vi "BuildTag.vi"(0 "Indent":i8=-1, 2 "tag":string, 3 "value":string, 4 "string in":string) -> (1 "string out":string)   [LabVIEW 2016]
doc: "Builds an XML string with tags"
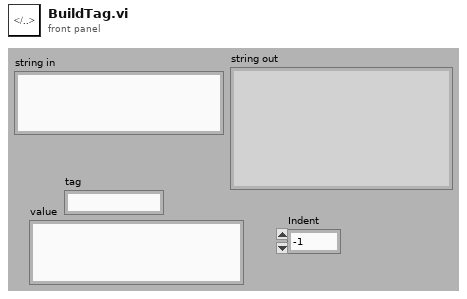
[diagram p1: front panel]
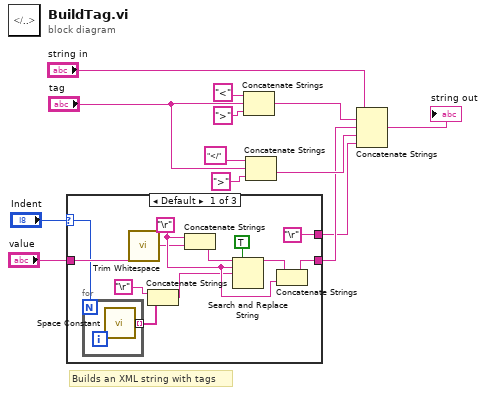
[diagram p0: block diagram]
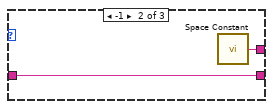
[diagram p2: hidden frame]
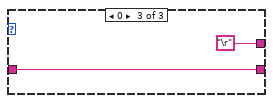
[diagram p3: hidden frame]
diagram:
  # "Builds an XML string with tags"
  n1 = case shown="Default" "Indent" {
    selector: "Indent" -> [w15 _ _]
    tunnel: [w23 w28 w30] -> w5
    tunnel: "value" -> [w20 w28 w30]
    tunnel: ["\r" w27 "\r"] -> w1
    frame Default {
      w22 = "\r"
      n2 = for {
        N: w15 -> [_]
        tunnel: [w26] -> w17 mode=indexing
        n3 = call "Space Constant.vi"() -> ("String"=w26:string)
      }
      n4 = call "Trim Whitespace.vi"("string"=w20) -> ("trimmed string"=w19:string)  [unwired: 1 in]
      n5 = Concatenate Strings("\r", w17) -> (w16:string)
      n6 = Concatenate Strings(w22, w19) -> (w21:string)
      n7 = Search and Replace String(replace all?=TRUE ("replace all? (F)"), input string=w21, search string=w22, replace string=w16) -> (result string=w24:string)  [unwired: 4 in, 3 out]
      n8 = Concatenate Strings(w24, w22) -> (w23:string)
    }
    frame -1 {
      n9 = call "Space Constant.vi"() -> ("String"=w27:string)
    }
    frame 0 {
    }
  }
  n10 = Concatenate Strings("<", "tag", ">") -> (w11:string)
  n11 = Concatenate Strings("</", "tag", ">") -> (w12:string)
  n12 = Concatenate Strings("string in", w11, w5, w12, w1) -> (→"string out":string)
